vi "TMCMonitor.vi"() -> ()   [LabVIEW 2019]
uses:
  Utility/Monitor Communication/Torque_TMC/TMCCluster.ctl
  Global/Global Variables/Data_Display_global.vi
  Instrument_Setup.vi
  <vilib>/Instr/_visa.llb/VISA Configure Serial Port (Serial Instr).vi
panel:
  out "error out":errorcluster
  in  "error in (no error)":errorcluster
  in  "stop":bool
  in  "TMC Cluster":T1
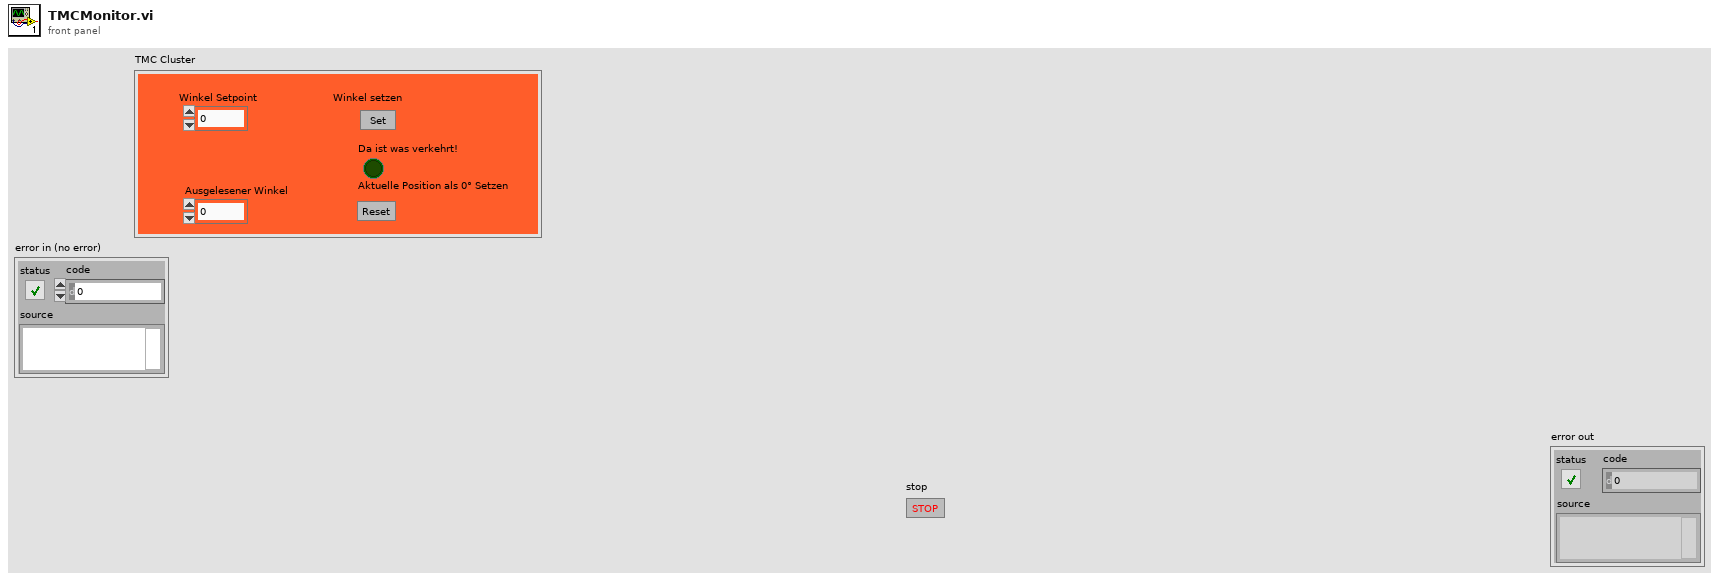
[diagram p1: front panel]
types:
  T1 = typedef "TMCCluster.ctl" = cluster{"Winkel Setpoint":dbl, "Ausgelesener Winkel":dbl, "Aktuelle Position als 0° Setzen":bool, "Da ist was verkehrt!":bool, "Winkel setzen":bool}
  T2 = typedef "TMC_Setup.ctl" = cluster{"flow control":u16, "stop bits":u16, "parity":u16, "data bits":u16, "baud rate":u32, "VISA Torque Motor":refnum<visa-resource-name>, "Set Angle through\ncommand file":bool}
  T3 = typedef "TMC_Control.ctl" = cluster{"Winkel Setpoint":dbl, "Aktuelle Position als 0° Setzen":bool, "Winkel setzen":bool}
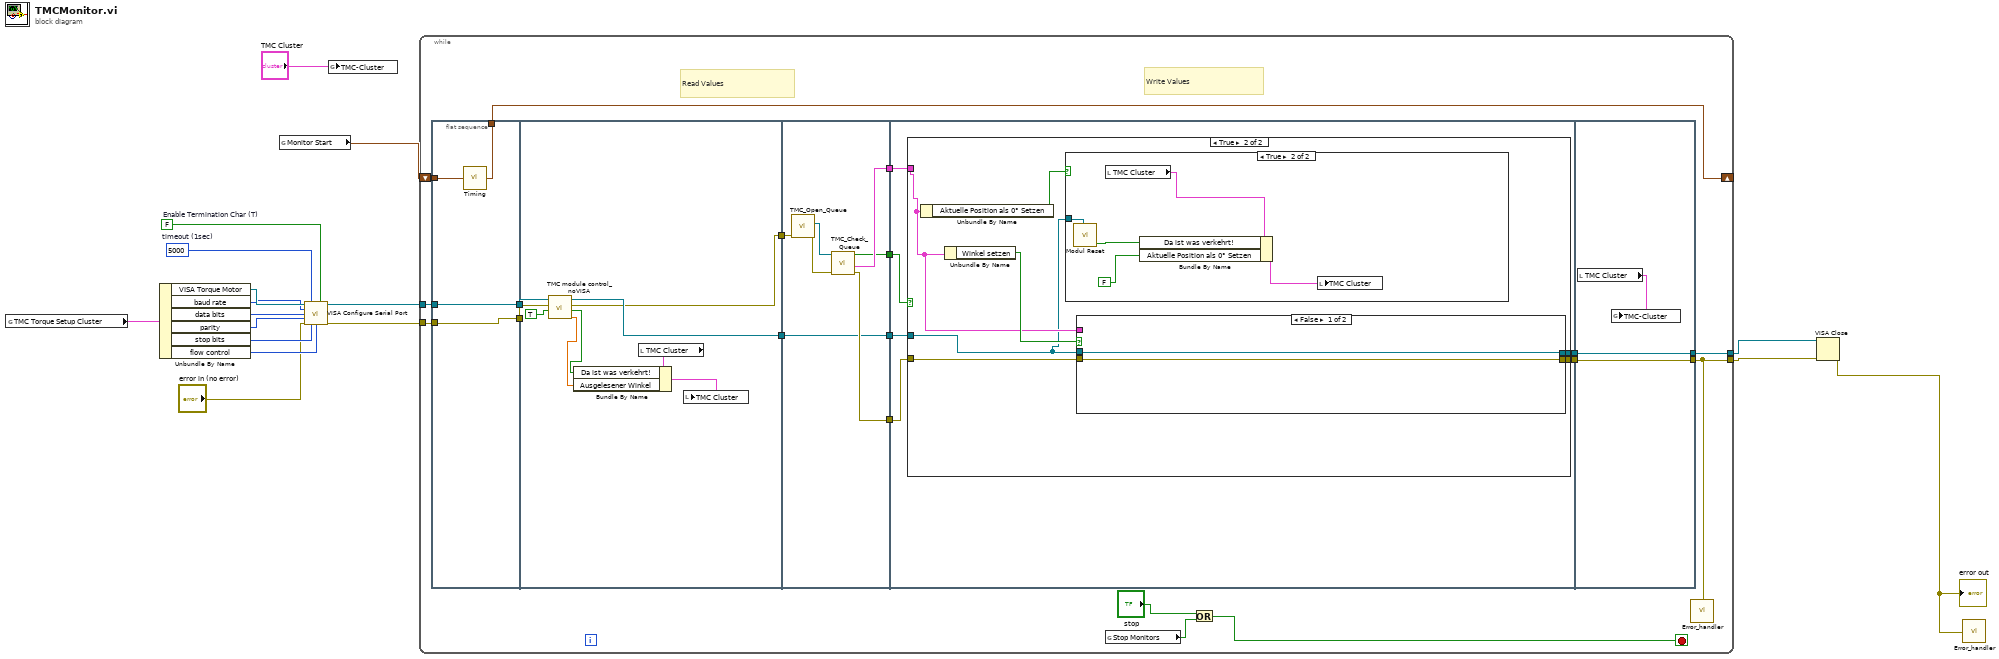
[diagram p0: block diagram]
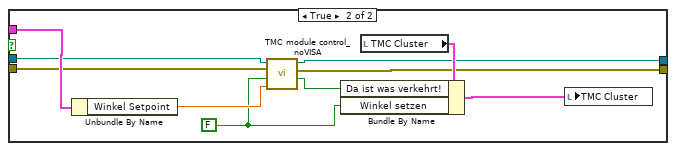
[diagram p3: hidden frame]
diagram:
  w5 = FALSE  # Enable Termination Char (T)
  w6 = u32 5000  # timeout (1sec)
  n1 = global read "Instrument_Setup.vi" "TMC Torque Setup Cluster"() -> (w14:T2)
  n2 = Unbundle By Name(w14) -> ("VISA Torque Motor"=w13:refnum<visa-resource-name>, "baud rate"=w12:u32, "data bits"=w11:u16, "parity"=w10:u16, "stop bits"=w9:u16, "flow control"=w8:u16)
  n3 = global read "Data_Display_global.vi" "Monitor Start"() -> (w16:timestamp)
  n4 = call-poly "VISA Configure Serial Port"("VISA resource name"=w13, "timeout (10sec)"=w6, "Enable Termination\nChar (T)"=w5, "baud rate (9600)"=w12, "data bits (8)"=w11, "parity (0:none)"=w10, "error in (no error)"="error in (no error)", "stop bits (10: 1 bit)"=w9, "flow control (0:none)"=w8) -> ("VISA resource name out"=w4:refnum<visa-resource-name>, "error out"=w3:errorcluster)  [unwired: 5 in]
  n5 = global write "Data_Display_global.vi" "TMC-Cluster"("TMC Cluster") -> ()
  n6 = while {
    shift-right: [w30] -> _
    shift-left: w16 -> [w31]
    tunnel: [w18] -> w1
    tunnel: w4 -> [w23]
    tunnel: w3 -> [w21]
    tunnel: [w19] -> w2
    stop <- w34 stop-if-true
    # "Write Values"
    # "Read Values"
    n7 = flat-sequence {
      tunnel: w31 -> [w40]
      tunnel: [w39] -> w30
      tunnel: [w38] -> w24
      tunnel: w23 -> [w38]
      tunnel: [w37] -> w22
      tunnel: w21 -> [w37]
      tunnel: [w43] -> w32
      tunnel: [w44] -> w28
      tunnel: w24 -> [w47]
      tunnel: w22 -> [w46]
      tunnel: [w54] -> w33
      tunnel: w32 -> [w53]
      tunnel: [w52] -> w29
      tunnel: w28 -> [w51]
      tunnel: [w51] -> w27
      tunnel: [w50] -> w25
      tunnel: w33 -> [w61]
      tunnel: w29 -> [w62]
      tunnel: w27 -> [w60]
      tunnel: [w59] -> w26
      tunnel: w25 -> [w58]
      tunnel: [w57] -> w20
      tunnel: [w90] -> w18
      tunnel: w26 -> [w90]
      tunnel: w20 -> [w89]
      tunnel: [w89] -> w19
      frame #0 {
        n8 = call "Timing.vi"("start time (s)"=w40) -> ("last reading (s)"=w39:timestamp)
      }
      frame #1 {
        n9 = call "TMC module control_noVISA.vi"("Nur Position auslesen"=TRUE, "error in (no error)"=w46, "VISA resource name"=w47) -> ("Ausgelesener Winkel [°]"=w41:dbl, "Fehler"=w42:bool, "error out"=w43:errorcluster, "VISA resource name out"=w44:refnum<visa-resource-name>)  [unwired: 5 in]
        n10 = local read "TMC Cluster"() -> (w49:T1)
        n11 = Bundle By Name(cluster=w49, "Da ist was verkehrt!"=w42, "Ausgelesener Winkel"=w41) -> (w48:T1)
        n12 = local write "TMC Cluster"(w48) -> ()
      }
      frame #2 {
        n13 = call "TMC_Open_Queue.vi"("error in (no error)"=w53) -> ("error out"=w55:errorcluster, "queue out"=w56:refnum<queue>)  [unwired: 9 in]
        n14 = call "TMC_Check_Queue.vi"("error in (no error)"=w55, "queue"=w56) -> ("error out"=w54:errorcluster, "TMC-Control"=w52:T3, "New Entries?"=w50:bool)  [unwired: 6 in]
      }
      frame #3 {
        n15 = case shown="True" w58 {
          tunnel: w62 -> [_ w69]
          tunnel: w61 -> [w63 w67]
          tunnel: w60 -> [w64 w65]
          tunnel: [w63 w68] -> w59
          tunnel: [w64 w66] -> w57
          frame False {
          }
          frame True {
            n16 = Unbundle By Name(w69) -> ("Aktuelle Position als 0° Setzen"=w71:bool)
            n17 = Unbundle By Name(w69) -> ("Winkel setzen"=w70:bool)
            n18 = case shown="True" w71 {
              tunnel: w65 -> [_ w84]
              frame False {
              }
              frame True {
                n19 = call "Modul Reset.vi"("VISA resource name"=w84) -> ("Fehler"=w87:bool)  [unwired: 9 in]
                n20 = local read "TMC Cluster"() -> (w86:T1)
                n21 = Bundle By Name(cluster=w86, "Da ist was verkehrt!"=w87, "Aktuelle Position als 0° Setzen"=FALSE) -> (w88:T1)
                n22 = local write "TMC Cluster"(w88) -> ()
              }
            }
            n23 = case shown="False" w70 {
              tunnel: w69 -> [_ w82]
              tunnel: w65 -> [w73 w80]
              tunnel: [w72 w78] -> w68
              tunnel: w67 -> [w72 w79]
              tunnel: [w73 w77] -> w66
              frame False {
              }
              frame True {
                w75 = FALSE
                n24 = Unbundle By Name(w82) -> ("Winkel Setpoint"=w76:dbl)
                n25 = call "TMC module control_noVISA.vi"("Winkel [°]"=w76, "Nur Position auslesen"=w75, "error in (no error)"=w79, "VISA resource name"=w80) -> ("Fehler"=w74:bool, "error out"=w78:errorcluster, "VISA resource name out"=w77:refnum<visa-resource-name>)  [unwired: 4 in, 1 out]
                n26 = local read "TMC Cluster"() -> (w81:T1)
                n27 = Bundle By Name(cluster=w81, "Da ist was verkehrt!"=w74, "Winkel setzen"=w75) -> (w83:T1)
                n28 = local write "TMC Cluster"(w83) -> ()
              }
            }
          }
        }
      }
      frame #4 {
        n29 = local read "TMC Cluster"() -> (w91:T1)
        n30 = global write "Data_Display_global.vi" "TMC-Cluster"(w91) -> ()
      }
    }
    n31 = global read "Data_Display_global.vi" "Stop Monitors"() -> (w35:bool)
    n32 = Or(x="stop", y=w35) -> (x .or. y?=w34:bool)
    n33 = call "Error_handler.vi"("error constant"=w18) -> ()
  }
  n34 = VISA Close(VISA resource name=w2, error in (no error)=w1) -> (error out=w15:errorcluster)
  "error out" <- w15
  n35 = call "Error_handler.vi"("error constant"=w15) -> ()
